vi "leer_serial.vi"() -> ()   [LabVIEW 2018]
uses:
  <vilib>/Instr/_visa.llb/VISA Configure Serial Port (Instr).vi
panel:
  out "*(type *) &x 2":u8
  out "*(type *) &x":string
  in  "stop":bool
  in  "baud rate (9600)":u32=9600
  in  "VISA resource name":refnum<visa-resource-name>
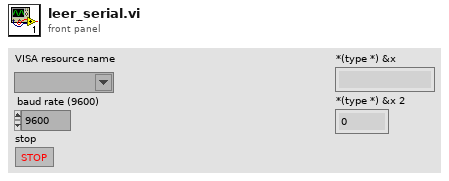
[diagram p1: front panel]
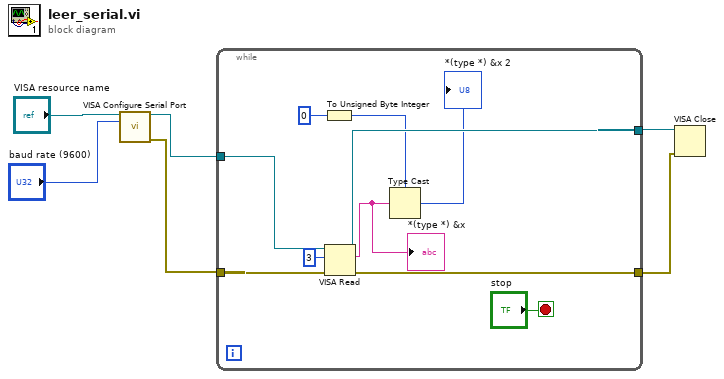
[diagram p0: block diagram]
diagram:
  n1 = call-poly "VISA Configure Serial Port"("VISA resource name"="VISA resource name", "baud rate (9600)"="baud rate (9600)") -> ("VISA resource name out"=w4:refnum<visa-resource-name>, "error out"=w2:errorcluster)  [unwired: 12 in]
  n2 = while {
    tunnel: w4 -> [w15]
    tunnel: [w14] -> w3
    tunnel: w2 -> [w11]
    tunnel: [w7] -> w1
    stop <- "stop" stop-if-true
    n3 = To Unsigned Byte Integer(number=u16 0) -> (unsigned 8bit integer=w10:u8)
    n4 = VISA Read(VISA resource name=w15, byte count=u32 3, error in (no error)=w11) -> (VISA resource name out=w14:refnum<visa-resource-name>, read buffer=w8:string, error out=w7:errorcluster)  [unwired: 1 out]
    "*(type *) &x" <- w8
    n5 = Type Cast(type=w10, x=w8) -> (*(type *) &x=→"*(type *) &x 2":u8)
  }
  n6 = VISA Close(VISA resource name=w3, error in (no error)=w1) -> ()  [unwired: 1 out]
